vi "Error - Log.vi"(8 "error in (no error)":errorcluster, 9 "Description":string, 10 "Date/Time":string, 11 "Level":T1) -> (0 "error out":errorcluster)   [LabVIEW 2017]
doc: "Maintain a log file with enhanced errors data.\n[Covers: EH4]"
uses:
  Controls/Error Level.ctl
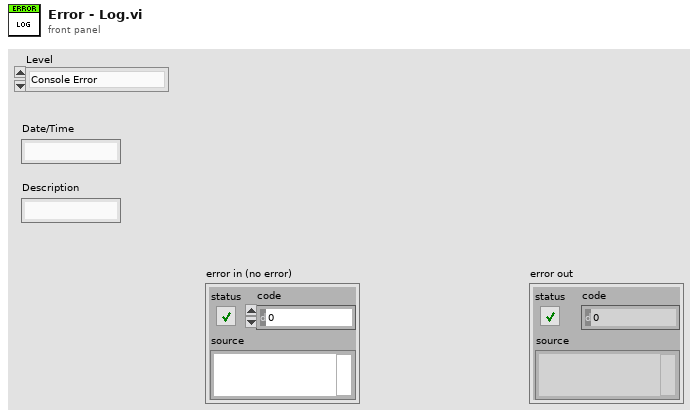
[diagram p1: front panel]
types:
  T1 = typedef "Error Level.ctl" = enum16{"Console Error", "Sensor Interface IO Error", "Process Step Error"}
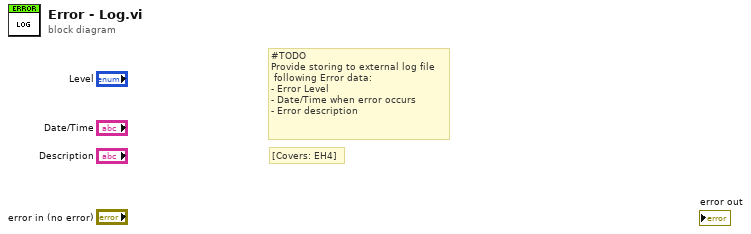
[diagram p0: block diagram]
diagram:
  # "[Covers: EH4]"
  # "#TODO\nProvide storing to external log file\n following Error data:\n- Error Level\n- Date/Time when error occurs\n- Error description"
